vi "iterationScanDone.vi"(8 "error in (no error)":errorcluster, 11 "Model in":refnum<class "Model.lvclass">) -> (0 "error out":errorcluster, 2 "Done?":bool, 3 "Model out":refnum<class "Model.lvclass">)   [LabVIEW 2015, in "Model.lvclass"]
uses:
  Model.lvclass
  Model.lvclass/Model.ctl
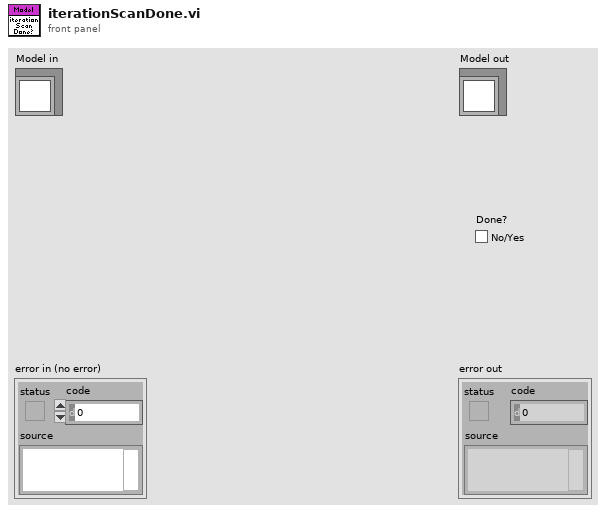
[diagram p1: front panel]
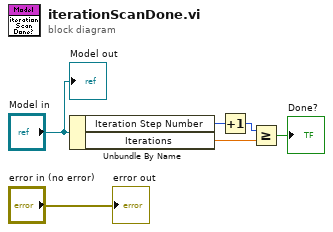
[diagram p0: block diagram]
diagram:
  n1 = Unbundle By Name("Model in") -> ("Iteration Step Number"=w4:u16, "Iterations"=w3:dbl)
  n2 = Increment(x=w4) -> (x+1=w2:u16)
  n3 = Greater Or Equal?(x=w2, y=w3) -> (x >= y?=→"Done?":bool)
  "error out" <- "error in (no error)"
  "Model out" <- "Model in"
